vi "CreateSolidBrush.vi"(8 "error in (no error)":errorcluster, 11 "ColorRef":refnum<k24>) -> (0 "error out":errorcluster, 3 "SolidBrushRef":refnum<k24>)   [LabVIEW 2020, in "LcPictureBox.lvclass"]
uses:
  LcPictureBox.lvclass
  System.Drawing
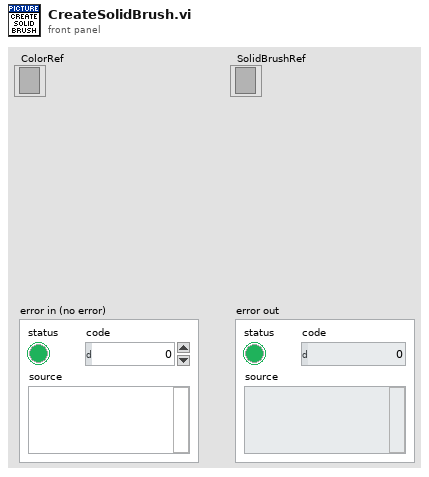
[diagram p1: front panel]
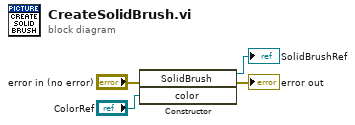
[diagram p0: block diagram]
diagram:
  n1 = constructor class="SolidBrush"(error in="error in (no error)", "color"="ColorRef") -> (reference out=→"SolidBrushRef":refnum<k24>, error out=→"error out":errorcluster)  [unwired: 2 in, 2 out]
